vi "Message.vi"(8 "error in (no error)":errorcluster, 11 "Board_Game in":refnum<class "Board_Game.lvclass">) -> (0 "error out":errorcluster)   [LabVIEW 2021, in "Board_Game.lvclass"]
uses:
  Board_Game.lvclass
  Board_Game.lvclass/Board_Game.ctl
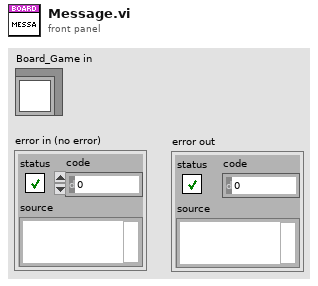
[diagram p1: front panel]
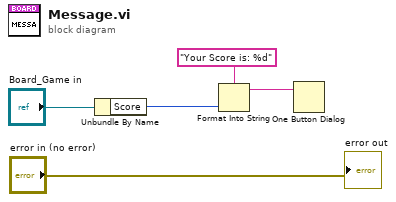
[diagram p0: block diagram]
diagram:
  n1 = Unbundle By Name("Board_Game in") -> ("Score"=w2:u32)
  n2 = Format Into String(format string="Your Score is: %d", w2) -> (resulting string=w4:string)  [unwired: 2 in, 1 out]
  n3 = One Button Dialog(message=w4) -> ()  [unwired: 1 in, 1 out]
  "error out" <- "error in (no error)"
